vi "tm_settrigger.vi"(8 "error in (no error)":errorcluster, 9 "Trigger Polarity":u32(ring)=1 items=["Negative"=1, "Positive"=2], 10 "Trigger Mode":u32(ring)=1 items=["Internal"=1, "External Edge"=2, "External Level"=4, "Software"=32, "Fast Repetition"=64, "TDI"=128, "Trigger Start"=512, "Sync Readout"=1024], 11 "Handle in":u32) -> (0 "error out":errorcluster, 3 "Handle out":u32)   [LabVIEW 2011]
uses:
  tmcamcon.dll
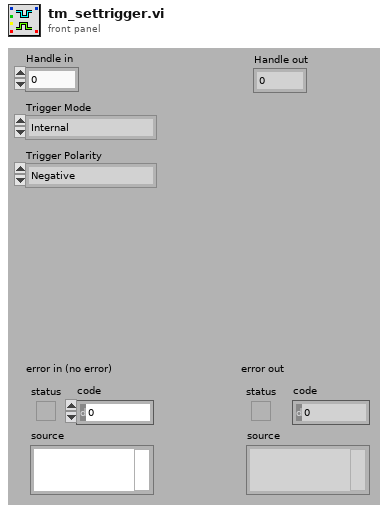
[diagram p1: front panel]
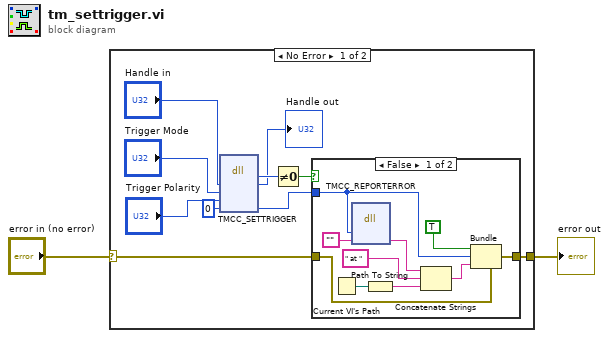
[diagram p0: block diagram]
diagram:
  n1 = case shown="No Error" "error in (no error)" {
    selector: "error in (no error)" -> [w4 w24]
    tunnel: [w3 w24] -> w1
    frame No Error {
      n2 = dll-call lib="tmcamcon.dll" fn="TMCC_SETTRIGGER"("HDCAM"="Handle in", "mode"="Trigger Mode", "polarity"="Trigger Polarity", "Erval"=0) -> (w12:u32, "HDCAM"=→"Handle out":i32, "Erval"=w5:i32)  [unwired: 5 in, 2 out]
      n3 = Not Equal To 0?(x=w12) -> (x != 0?=w6:bool)
      n4 = case shown="False" w6 {
        tunnel: w4 -> [w22 w23]
        tunnel: [w21 w23] -> w3
        tunnel: w5 -> [w15 _]
        frame False {
          n5 = Current VI's Path() -> (path=w20:path)
          n6 = dll-call lib="tmcamcon.dll" fn="TMCC_REPORTERROR"("error"=w15, "buf"="") -> ("buf"=w14:string)  [unwired: 5 in, 2 out]
          n7 = Path To String(path=w20) -> (string=w16:string)
          n8 = Concatenate Strings(w14, " at ", w16) -> (w19:string)
          n9 = Bundle(cluster=w22, "status"=TRUE, "code"=w15, "source"=w19) -> (w21:errorcluster)
        }
        frame True {
        }
      }
    }
    frame Error {
    }
  }
  "error out" <- w1
